vi "LookupTable.vi"(10 "element":dbl) -> (2 "element 2":dbl)   [LabVIEW 2011]
panel:
  in  "array":dbl[][](array[numeric])
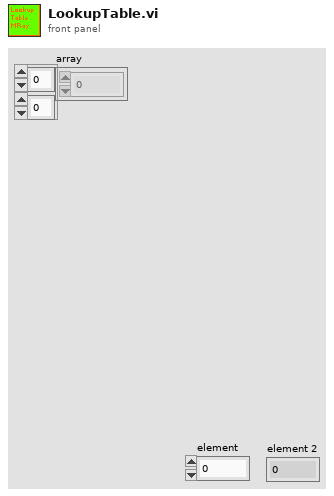
[diagram p1: front panel]
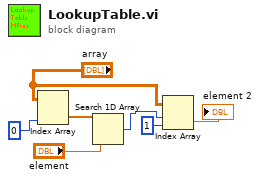
[diagram p0: block diagram]
diagram:
  n1 = Index Array(array="array", index (col)=0 ("disabled index (col)")) -> (element=w6:dbl[])  [unwired: 1 in]
  n2 = Search 1D Array(1D array=w6, element="element") -> (index of element=w3:i32)  [unwired: 1 in]
  n3 = Index Array(array="array", index (row)=w3, index (col)=1) -> (element=→"element 2":dbl)
